vi "UnFormat Packet Bytes.vi"(11 "spreadsheet string":string) -> (3 "array":u8[](array[numeric]))   [LabVIEW 2025, in "Automotive Ethernet Bus Monitor UI.lvlib"]
uses:
  Automotive Ethernet Bus Monitor UI.lvlib
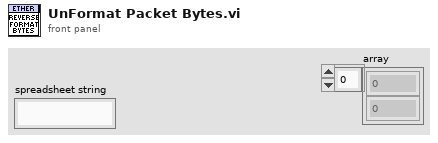
[diagram p1: front panel]
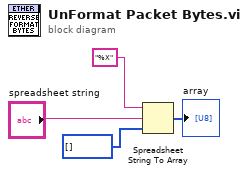
[diagram p0: block diagram]
diagram:
  n1 = Spreadsheet String To Array(format string="%X", spreadsheet string="spreadsheet string", array type (2D Dbl)=u8[] []) -> (array=→"array":u8[])  [unwired: 1 in]
